vi "CalculateDose.vi"(9 "Period (sec)":dbl, 10 "DPA Rate":dbl, 11 "Dose In (DPA)":dbl) -> (3 "Dose Out (DPA)":dbl)   [LabVIEW 2012]
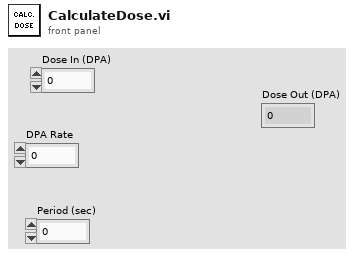
[diagram p1: front panel]
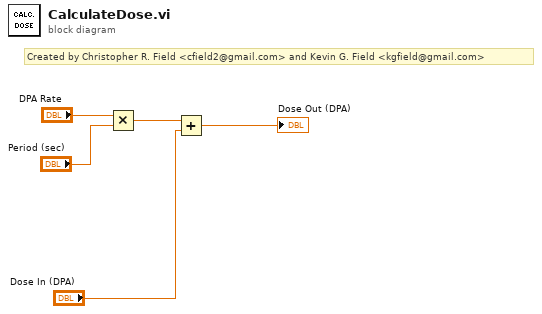
[diagram p0: block diagram]
diagram:
  # "Created by Christopher R. Field <cfield2@gmail.com> and Kevin G. Field <kgfield@gmail.com>"
  n1 = Multiply(x="DPA Rate", y="Period (sec)") -> (x*y=w3:dbl)
  n2 = Add(x=w3, y="Dose In (DPA)") -> (x+y=→"Dose Out (DPA)":dbl)
